vi "DO Create Channel.vi"(8 "error in (no error)":errorcluster, 10 "Digital Configuration":T1, 11 "Mech Pump in":refnum<class "Mech Pump.lvclass">) -> (0 "error out":errorcluster, 3 "Mech Pump out":refnum<class "Mech Pump.lvclass">)   [LabVIEW 2021, in "Mech Pump.lvlib" / "Mech Pump.lvclass"]
uses:
  Mech Pump.lvclass
  Mech Pump.lvclass/Mech Pump.ctl
  DAQ-arch/Digital Output On Demand/Digital Output On Demand/Digital Output On Demand.lvclass
  DAQ-arch/Digital Configure.ctl
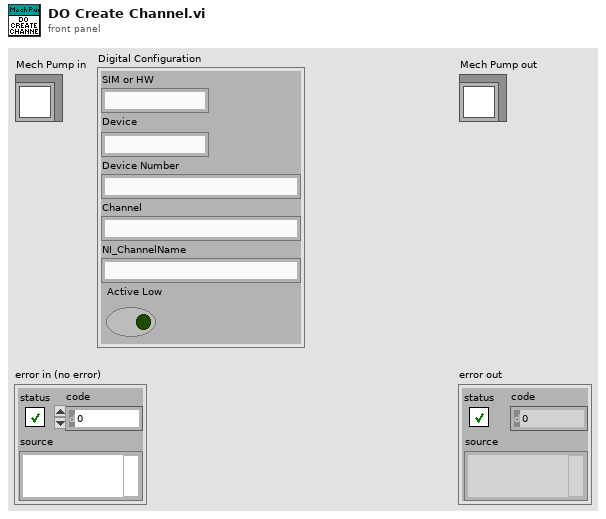
[diagram p1: front panel]
types:
  T1 = typedef "Digital Configure.ctl" = cluster{"SIM or HW":string, "Device":string, "Device Number":string, "Channel":string, "NI_ChannelName":string, "Active Low":bool}
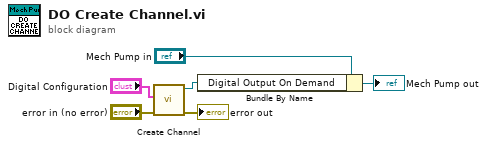
[diagram p0: block diagram]
diagram:
  n1 = call "Create Channel.vi"("error in (no error)"="error in (no error)", "Digital Configuration"="Digital Configuration") -> ("error out"=→"error out":errorcluster, "Digital Output On Demand out"=w4:refnum<class "Digital Output On Demand.lvclass">)  [unwired: 8 in]
  n2 = Bundle By Name(cluster="Mech Pump in", "Digital Output On Demand"=w4) -> (→"Mech Pump out":refnum<class "Mech Pump.lvclass">)
